vi "DUMMY.vi"() -> ()   [LabVIEW 2020]
uses:
  <vilib>/Waveform/WDTOps.llb/WDT Waveform Duration DBL.vi
  <vilib>/Waveform/WDTOps.llb/WDT Get Waveform Subset DBL.vi
  <vilib>/measure/mamon.llb/Trigger Detection for 1 Channel.vi
  <vilib>/measure/NI_MAPro.lvlib
  <vilib>/measure/mascope.llb/Transition Measurements 1 chan.vi
panel:
  out "error out":errorcluster
  out "file path (OUT)":path
  in  "Request #":string
  in  "Project #":string
  in  "TEST #":string
  out "DONE Tdon":bool
  in  "Decision ?":bool
  out "Tdon (ns) (after filter)":dbl
  out "Cursor a : Channel 2 (after filter)":dbl
  out "Cursor a : Channel 1 (after filter)":dbl
  in  "ICE":dbl
  in  "VGE":dbl
  out "10% Vge (Theory)":dbl
  out "10% Ice (Theory)":dbl
  out "measurement info (CH2) \n(after filter)":T1 {"ref levels"."ref units" items=["absolute", "relative"]; "ref levels"."high ref level" format="%.2p"; "ref levels"."low ref level" format="%.2p"; "ref levels"."mid ref level" format="%.2p"; "end time" format="%.6e"; "start time" format="%.6e"}
  in  "reference  levels (CH2 initialize) (after filter)":T2={"high ref level"=90.0, "mid ref level"=50.0, "low ref level"=10.0, "ref units"=1} {"ref units" items=["absolute", "percent"]; "high ref level" format="%0.2f"; "low ref level" format="%0.2f"; "mid ref level" format="%0.2f"}
  out "measurement info (CH1) \n(after filter)":T1 {"ref levels"."ref units" items=["absolute", "relative"]; "ref levels"."high ref level" format="%.2p"; "ref levels"."low ref level" format="%.2p"; "ref levels"."mid ref level" format="%.2p"; "end time" format="%.6e"; "start time" format="%.6e"}
  in  "reference  levels (CH1 initialize) (after filter)":T2={"high ref level"=90.0, "mid ref level"=50.0, "low ref level"=10.0, "ref units"=1} {"ref units" items=["absolute", "percent"]; "high ref level" format="%0.2f"; "low ref level" format="%0.2f"; "mid ref level" format="%0.2f"}
  out "Waveform Graph":waveform(dbl)[](graph)
  out "Tdon after Noise Filter":waveform(dbl)[](graph) caption="Tdon (ns)"
  in  "error in (no error)":errorcluster
  in  "file path (IN)":path
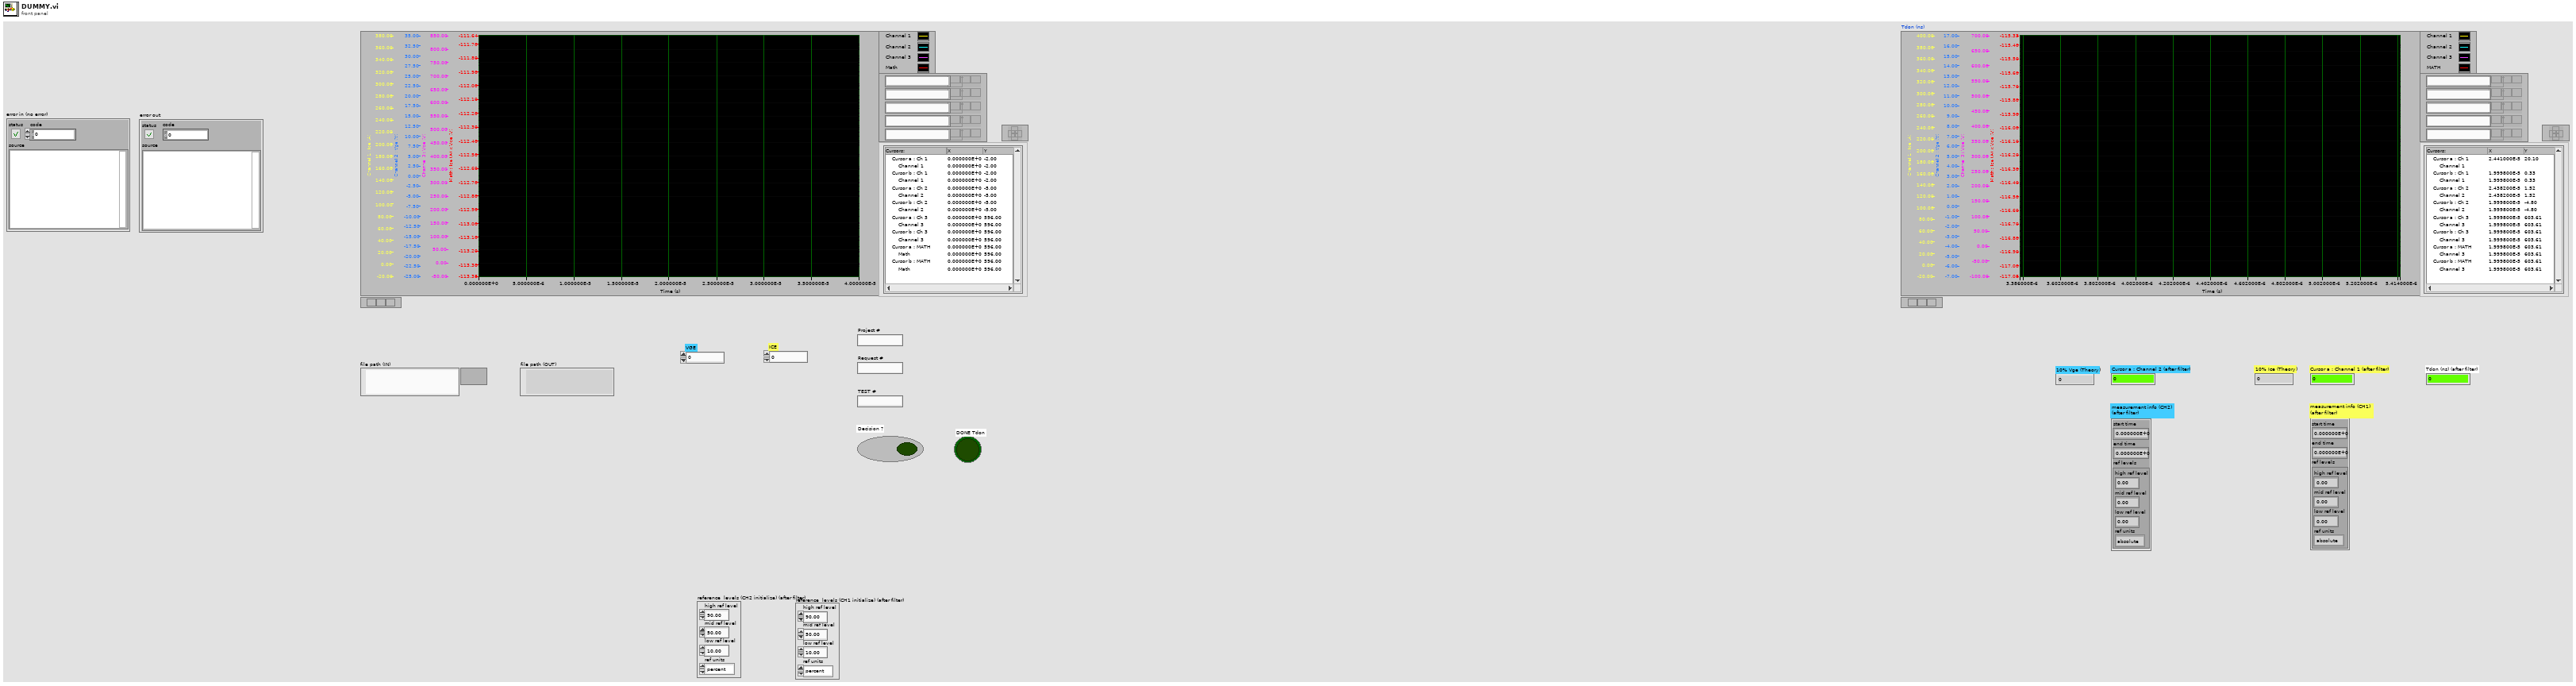
[diagram p1: front panel]
types:
  T1 = cluster{"start time":dbl, "end time":dbl, "ref levels":cluster{"high ref level":dbl, "mid ref level":dbl, "low ref level":dbl, "ref units":u16}}
  T2 = cluster{"high ref level":dbl, "mid ref level":dbl, "low ref level":dbl, "ref units":u16}
  T3 = enum32{"Invalid", "Standard", "Closed", "Hidden", "Minimized", "Maximized"}
  T4 = typedef "imagedata.ctl" = cluster{"image type":i32, "image depth":i32, "image":u8[], "mask":u8[], "colors":u32[], "Rectangle":cluster{"left":i16, "top":i16, "right":i16, "bottom":i16}}
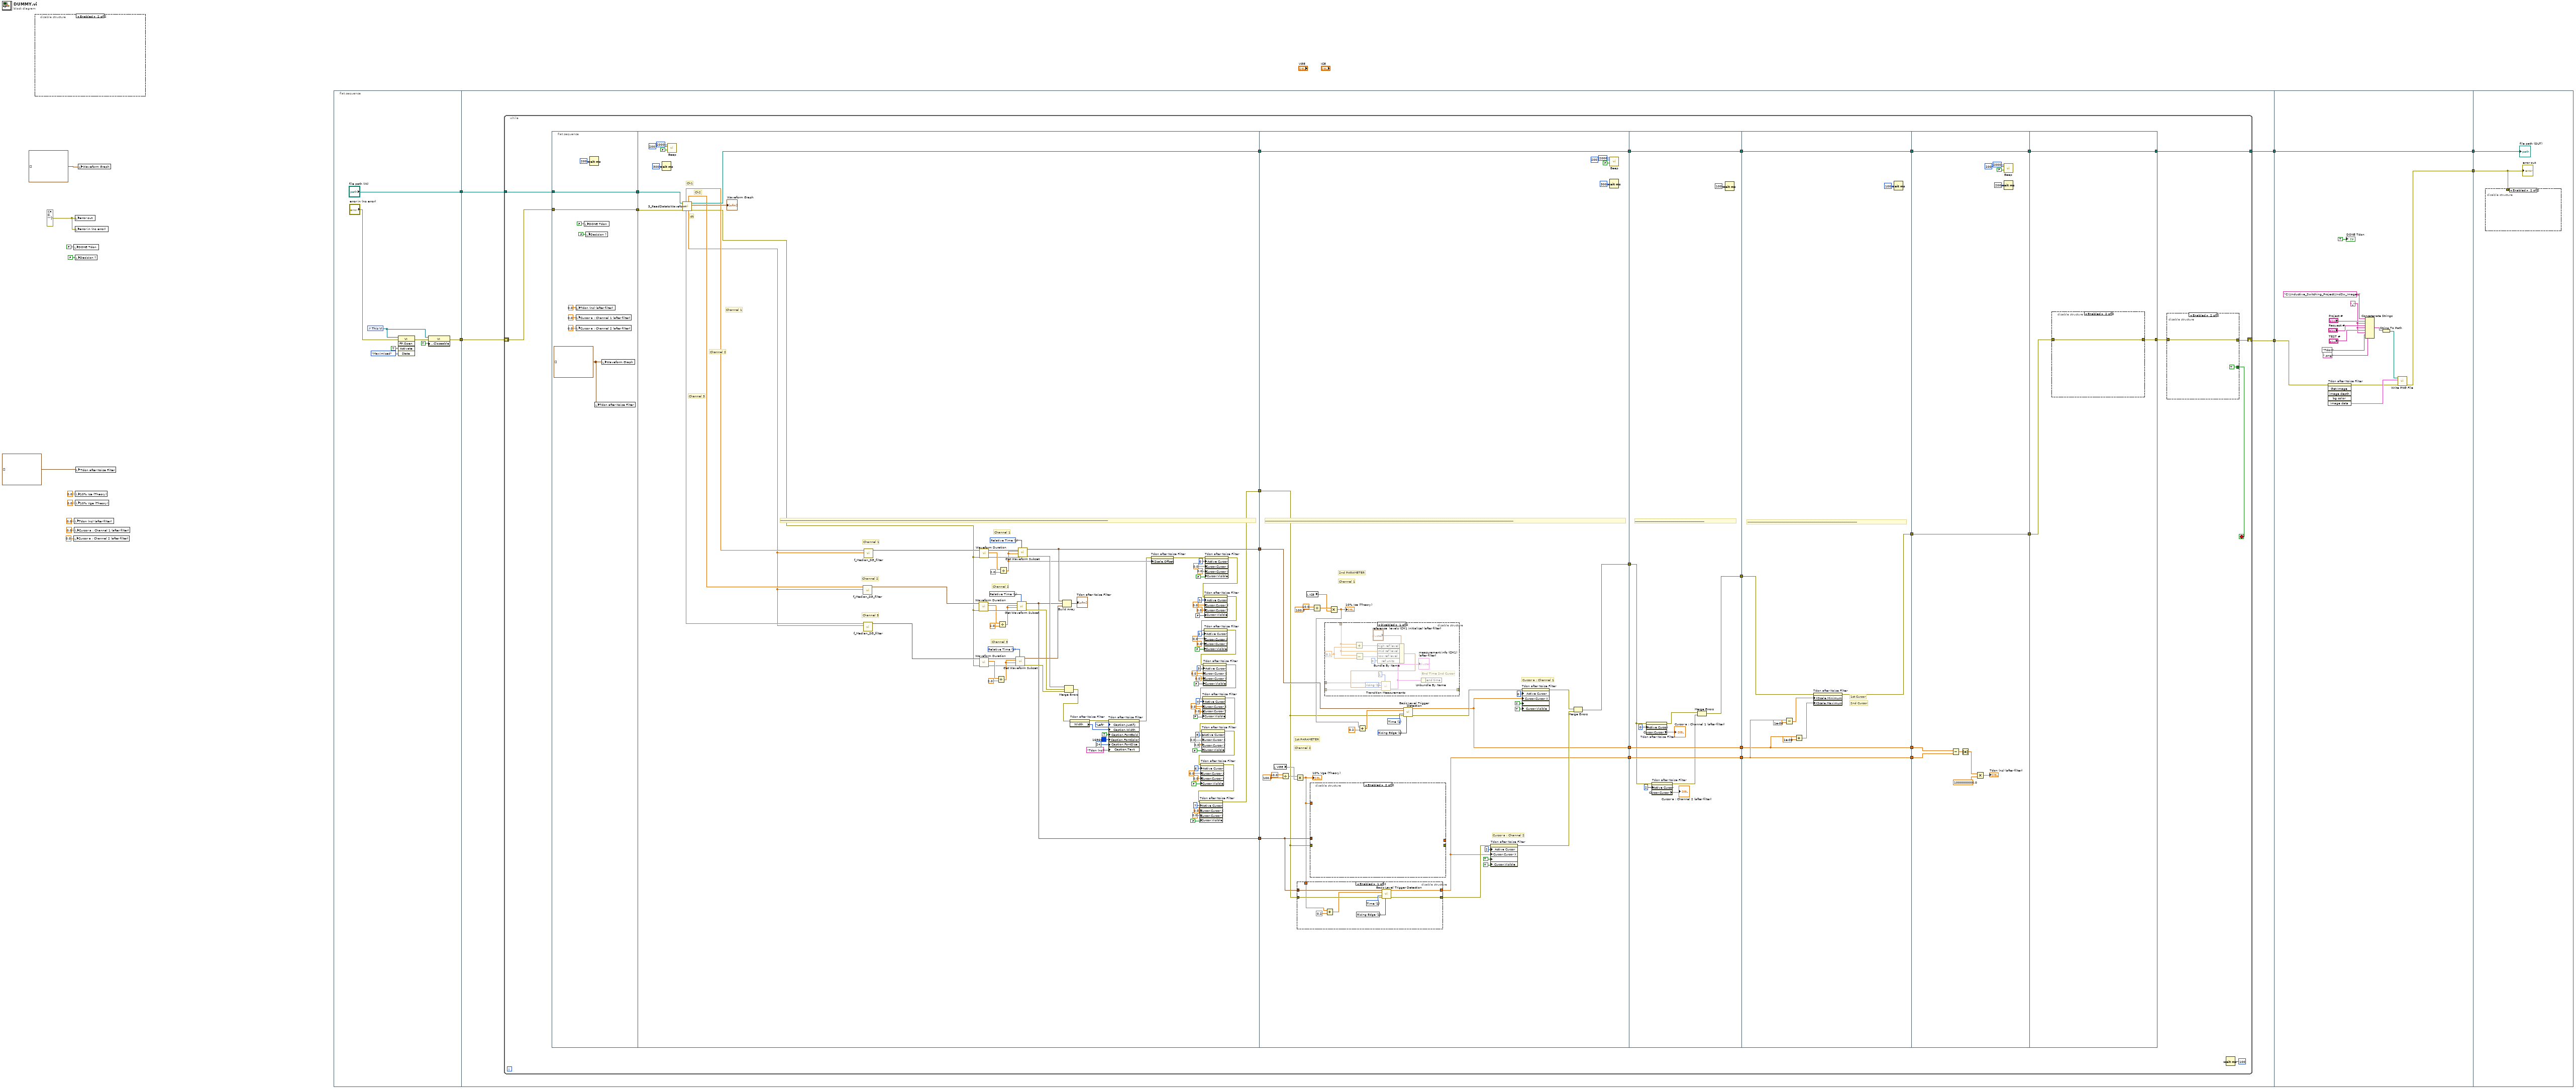
[diagram p0: block diagram]
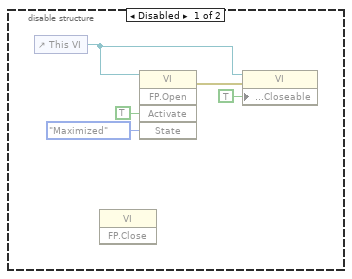
[diagram p2: hidden frame]
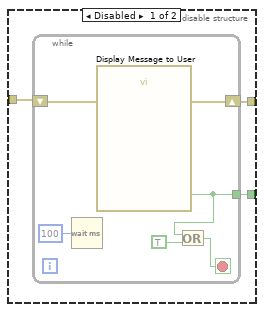
[diagram p3: hidden frame]
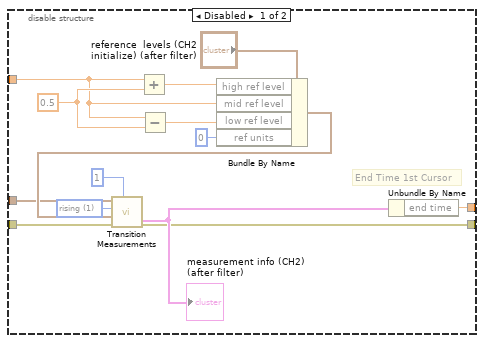
[diagram p6: hidden frame]
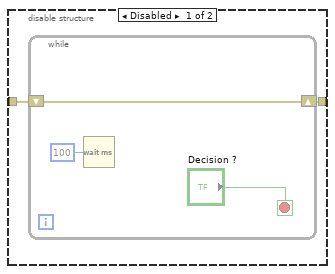
[diagram p7: hidden frame]
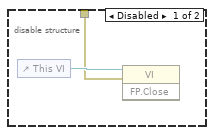
[diagram p8: hidden frame]
diagram:
  w9 = errorcluster {"status"=FALSE, "code"=0, "source"=""} ("error out")
  n1 = disable-structure shown="Enabled" {
    frame Disabled {
      n2 = control-ref of="This VI"() -> (w18:refnum<vi>)
      n3 = invoke class="VI" method="FP.Close"() -> (reference=w17:refnum<vi>)  [unwired: 2 in, 3 out]
      n4 = invoke class="VI" method="FP.Open"(reference=w18, "Activate"=TRUE ("Activate?"), "State"=T3."Maximized") -> (error in=w21:errorcluster, error out=w19:errorcluster)  [unwired: 1 in, 4 out]
      n5 = property class="VI"(reference=w18, error in=w19, "Front Panel.Closeable"=TRUE ("Front Panel Window:Closeable")) -> ()  [unwired: 2 out]
    }
    frame Enabled {
    }
  }
  n6 = local write "DONE Tdon"(FALSE ("DONE Tdon")) -> ()
  n7 = local write "Cursor a : Channel 2 (after filter)"(0.0 ("Cursor a : Channel 2 (after filter)")) -> ()
  n8 = local write "Tdon (ns) (after filter)"(0.0 ("Tdon (ns) (after filter)")) -> ()
  n9 = local write "Cursor a : Channel 1 (after filter)"(0.0 ("Cursor a : Channel 1 (after filter)")) -> ()
  n10 = local write "error out"(w9) -> ()
  n11 = local write "error in (no error)"(w9) -> ()
  n12 = local write "Decision ?"(FALSE ("Decision ?")) -> ()
  n13 = local write "10% Ice (Theory)"(0.0 ("10% Ice (Theory)")) -> ()
  n14 = local write "10% Vge (Theory)"(0.0 ("10% Vge (Theory)")) -> ()
  n15 = local write "Tdon after Noise Filter"(waveform(dbl)[] [] ("Tdon after Noise Filter")) -> ()
  n16 = local write "Waveform Graph"(waveform(dbl)[] [] ("Waveform Graph")) -> ()
  n17 = flat-sequence {
    tunnel: ["file path (IN)"] -> w16
    tunnel: [w26] -> w15
    tunnel: [w34] -> w14
    tunnel: [w33] -> w13
    tunnel: w16 -> [w35]
    tunnel: w15 -> [w32]
    tunnel: w14 -> [w289]
    tunnel: [w292] -> w12
    tunnel: [w291] -> w11
    tunnel: w13 -> [w291]
    tunnel: w12 -> [w303]
    tunnel: w11 -> [w304]
    frame #0 {
      n18 = control-ref of="This VI"() -> (w30:refnum<vi>)
      n19 = invoke class="VI" method="FP.Open"(reference=w30, error in="error in (no error)", "Activate"=TRUE ("Activate?"), "State"=T3."Maximized") -> (error out=w31:errorcluster)  [unwired: 1 in, 4 out]
      n20 = property class="VI"(reference=w30, error in=w31, "Front Panel.Closeable"=TRUE ("Front Panel Window:Closeable")) -> (error out=w26:errorcluster)  [unwired: 1 out]
    }
    frame #1 {
      n21 = while {
        tunnel: w35 -> [w58]
        shift-right: [w38] -> w34
        shift-left: w32 -> [w56]
        tunnel: [w54] -> w33
        stop <- w37 stop-if-true
        n22 = flat-sequence {
          tunnel: [w81] -> w62
          tunnel: [w82] -> w61
          tunnel: w58 -> [w82]
          tunnel: w56 -> [w81]
          tunnel: w62 -> [w173]
          tunnel: w61 -> [w171]
          tunnel: [w167] -> w60
          tunnel: [w141] -> w50
          tunnel: [w86] -> w49
          tunnel: [w83] -> w36
          tunnel: w60 -> [w205]
          tunnel: [w205] -> w53
          tunnel: w50 -> [w183]
          tunnel: w49 -> [w177]
          tunnel: [w188] -> w48
          tunnel: [w181] -> w47
          tunnel: [w174] -> w46
          tunnel: w36 -> [w187]
          tunnel: w53 -> [w256]
          tunnel: [w256] -> w52
          tunnel: w48 -> [w245]
          tunnel: w47 -> [w253]
          tunnel: w46 -> [w252]
          tunnel: [w253] -> w45
          tunnel: [w252] -> w44
          tunnel: [w246] -> w43
          tunnel: w52 -> [w266]
          tunnel: [w266] -> w59
          tunnel: w45 -> [w259]
          tunnel: w44 -> [w262]
          tunnel: w43 -> [w257]
          tunnel: [w262] -> w42
          tunnel: [w259] -> w41
          tunnel: [w258] -> w39
          tunnel: w59 -> [w275]
          tunnel: [w275] -> w55
          tunnel: w42 -> [w269]
          tunnel: w41 -> [w270]
          tunnel: [w267] -> w40
          tunnel: w39 -> [w267]
          tunnel: [w279] -> w51
          tunnel: w55 -> [w281]
          tunnel: [w281] -> w54
          tunnel: w40 -> [w280]
          frame #0 {
            w77 = waveform(dbl)[] [] ("Waveform Graph")
            n23 = local write "Tdon (ns) (after filter)"(0.0 ("Tdon (ns) (after filter)")) -> ()
            n24 = local write "Cursor a : Channel 1 (after filter)"(0.0 ("Cursor a : Channel 1 (after filter)")) -> ()
            n25 = local write "Cursor a : Channel 2 (after filter)"(0.0 ("Cursor a : Channel 2 (after filter)")) -> ()
            n26 = local write "DONE Tdon"(FALSE ("DONE Tdon")) -> ()
            n27 = local write "Decision ?"(FALSE ("Decision ?")) -> ()
            n28 = Wait (ms)(milliseconds to wait=u32 200) -> ()  [unwired: 1 out]
            n29 = local write "Tdon after Noise Filter"(w77) -> ()
            n30 = local write "Waveform Graph"(w77) -> ()
          }
          frame #1 {
            w162 = u16 1 items=["Samples", "Relative Time"] ("start/duration format")
            w151 = u16 1 items=["Samples", "Relative Time"] ("start/duration format")
            w150 = u16 1 items=["Samples", "Relative Time"] ("start/duration format")
            # "--------------------------------------------------------------------------------------------------------------------------------------------------------------------------------------------------------------------------------------------------------------------------------------------------------------------------------------"
            # "Channel 1"
            # "Channel 3"
            # "Channel 2"
            # "Channel 3"
            # "Channel 2"
            # "Channel 1"
            # "Channel 3"
            # "Channel 2"
            # "Channel 1"
            # "dt"
            # "Ch2"
            # "Ch1"
            n31 = Wait (ms)(milliseconds to wait=u32 300) -> ()  [unwired: 1 out]
            n32 = call <vilib>:"Beep.vi"("use system alert? (T)"=FALSE, "duration (msec)"=u32 200, "frequency (Hz)"=u32 2000) -> ()  [unwired: 9 in]
            n33 = call "3_ReadDatatoWaveform.vi"("error in (no error)"=w173, "file path (IN)"=w171) -> ("error out"=w84:errorcluster, "Waveform Graph"=→"Waveform Graph":waveform(dbl)[], "file path (OUT)"=w167:path, "dt"=w85:dbl, "Ch 2 Data"=w164:dbl[], "Ch 3 Data"=w163:dbl[], "Ch 1 Data"=w165:dbl[])  [unwired: 3 in]
            n34 = call "f_Median_SG_filter.vi"("dt"=w85, "Y"=w164) -> ("output waveform"=w144:waveform(dbl))  [unwired: 9 in]
            n35 = call "f_Median_SG_filter.vi"("dt"=w85, "Y"=w163) -> ("output waveform"=w143:waveform(dbl))  [unwired: 9 in]
            n36 = call "f_Median_SG_filter.vi"("dt"=w85, "Y"=w165) -> ("output waveform"=w145:waveform(dbl))  [unwired: 9 in]
            n37 = call-poly <vilib>:"Waveform Duration.vi"("error in (no error)"=w84, "waveform in"=w144) -> ("error out"=w156:errorcluster, "duration"=w153:dbl, "waveform out"=w155:waveform(dbl))  [unwired: 7 in]
            n38 = call-poly <vilib>:"Waveform Duration.vi"("error in (no error)"=w84, "waveform in"=w143) -> ("error out"=w157:errorcluster, "duration"=w160:dbl, "waveform out"=w158:waveform(dbl))  [unwired: 7 in]
            n39 = call-poly <vilib>:"Waveform Duration.vi"("error in (no error)"=w84, "waveform in"=w145) -> ("error out"=w146:errorcluster, "duration"=w149:dbl, "waveform out"=w147:waveform(dbl))  [unwired: 7 in]
            n40 = Divide(x=w160, y=2.0) -> (x/y=w161:dbl)
            n41 = Divide(x=w153, y=2.0) -> (x/y=w152:dbl)
            n42 = Divide(x=w149, y=2.0) -> (x/y=w128:dbl)
            n43 = call-poly <vilib>:"Get Waveform Subset.vi"("start/duration format"=w162, "error in (no error)"=w157, "duration"=w161, "start samples/time"=w161, "waveform in"=w158) -> ("error out"=w137:errorcluster, "waveform out"=w140:waveform(dbl))  [unwired: 1 in, 2 out]
            n44 = call-poly <vilib>:"Get Waveform Subset.vi"("start/duration format"=w151, "error in (no error)"=w156, "duration"=w152, "start samples/time"=w152, "waveform in"=w155) -> ("error out"=w138:errorcluster, "waveform out"=w83:waveform(dbl))  [unwired: 1 in, 2 out]
            n45 = call-poly <vilib>:"Get Waveform Subset.vi"("start/duration format"=w150, "error in (no error)"=w146, "duration"=w128, "start samples/time"=w128, "waveform in"=w147) -> ("error out"=w139:errorcluster, "waveform out"=w141:waveform(dbl))  [unwired: 1 in, 2 out]
            n46 = Build Array(w141, w83, w140) -> (→"Tdon after Noise Filter":waveform(dbl)[])
            n47 = Merge Errors(w139, w138, w137) -> (w136:errorcluster)
            n48 = property on="Tdon after Noise Filter" class="WFGraph (strict)"(error in=w136) -> (error out=w130:errorcluster, "Width"=w129:u32)  [unwired: 1 in, 1 out]
            n49 = property on="Tdon after Noise Filter" class="WFGraph (strict)"(error in=w130, "Caption.Justify"=enum16{"Left", "Center", "Right"}."Left" ("Caption.Justification"), "Caption.Width"=w129, "Caption.FontBold"=TRUE ("Caption.Font:Bold"), "Caption.FontColor"=u32 16860 ("Caption.Font:Color"), "Caption.FontSize"=u32 24 ("Caption.Font:Size"), "Caption.Text"="Tdon (ns)") -> (error out=w127:errorcluster)  [unwired: 1 in, 1 out]
            n50 = property on="Tdon after Noise Filter" class="WFGraph (strict)"(error in=w127, "XScale.Offset"=w128) -> (error out=w94:errorcluster)  [unwired: 1 in, 1 out]
            n51 = property on="Tdon after Noise Filter" class="WFGraph (strict)"(error in=w94, "Active Cursor"=u32 0, "Cursor.Cursor X"=0.0 ("Cursor.Cursor Position:Cursor X"), "Cursor.Cursor Y"=0.0 ("Cursor.Cursor Position:Cursor Y"), "Cursor.Visible"=FALSE) -> (error out=w93:errorcluster)  [unwired: 1 in, 1 out]
            n52 = property on="Tdon after Noise Filter" class="WFGraph (strict)"(error in=w93, "Active Cursor"=u32 1, "Cursor.Cursor X"=0.0 ("Cursor.Cursor Position:Cursor X"), "Cursor.Cursor Y"=0.0 ("Cursor.Cursor Position:Cursor Y"), "Cursor.Visible"=FALSE) -> (error out=w92:errorcluster)  [unwired: 1 in, 1 out]
            n53 = property on="Tdon after Noise Filter" class="WFGraph (strict)"(error in=w92, "Active Cursor"=u32 2, "Cursor.Cursor X"=0.0 ("Cursor.Cursor Position:Cursor X"), "Cursor.Cursor Y"=0.0 ("Cursor.Cursor Position:Cursor Y"), "Cursor.Visible"=FALSE) -> (error out=w91:errorcluster)  [unwired: 1 in, 1 out]
            n54 = property on="Tdon after Noise Filter" class="WFGraph (strict)"(error in=w91, "Active Cursor"=u32 3, "Cursor.Cursor X"=0.0 ("Cursor.Cursor Position:Cursor X"), "Cursor.Cursor Y"=0.0 ("Cursor.Cursor Position:Cursor Y"), "Cursor.Visible"=FALSE) -> (error out=w90:errorcluster)  [unwired: 1 in, 1 out]
            n55 = property on="Tdon after Noise Filter" class="WFGraph (strict)"(error in=w90, "Active Cursor"=u32 4, "Cursor.Cursor X"=0.0 ("Cursor.Cursor Position:Cursor X"), "Cursor.Cursor Y"=0.0 ("Cursor.Cursor Position:Cursor Y"), "Cursor.Visible"=FALSE) -> (error out=w89:errorcluster)  [unwired: 1 in, 1 out]
            n56 = property on="Tdon after Noise Filter" class="WFGraph (strict)"(error in=w89, "Active Cursor"=u32 5, "Cursor.Cursor X"=0.0 ("Cursor.Cursor Position:Cursor X"), "Cursor.Cursor Y"=0.0 ("Cursor.Cursor Position:Cursor Y"), "Cursor.Visible"=FALSE) -> (error out=w88:errorcluster)  [unwired: 1 in, 1 out]
            n57 = property on="Tdon after Noise Filter" class="WFGraph (strict)"(error in=w88, "Active Cursor"=u32 6, "Cursor.Cursor X"=0.0 ("Cursor.Cursor Position:Cursor X"), "Cursor.Cursor Y"=0.0 ("Cursor.Cursor Position:Cursor Y"), "Cursor.Visible"=FALSE) -> (error out=w87:errorcluster)  [unwired: 1 in, 1 out]
            n58 = property on="Tdon after Noise Filter" class="WFGraph (strict)"(error in=w87, "Active Cursor"=u32 7, "Cursor.Cursor X"=0.0 ("Cursor.Cursor Position:Cursor X"), "Cursor.Cursor Y"=0.0 ("Cursor.Cursor Position:Cursor Y"), "Cursor.Visible"=FALSE) -> (error out=w86:errorcluster)  [unwired: 1 in, 1 out]
          }
          frame #2 {
            w184 = u16 1 items=["Falling Edge", "Rising Edge"] ("trigger slope")
            w185 = u16 1 items=["Index", "Time"] ("location mode")
            # "Cursor a : Channel 1"
            # "2nd PARAMETER"
            # "Channel 1"
            # "Cursor a : Channel 2"
            # "1st PARAMETER"
            # "Channel 2"
            # "-------------------------------------------------------------------------------------------------------------------------------------------------------------------------------------------------------------------------------------------------------"
            n59 = local read "VGE"() -> (w186:dbl)
            n60 = Divide(x=10.0, y=100.0) -> (x/y=w202:dbl)
            n61 = Multiply(x=w202, y=w186) -> (x*y=w176:dbl)
            "10% Vge (Theory)" <- w176
            n62 = disable-structure shown="Enabled" {
              disable-tunnel: [w217 _] -> w174
              disable-tunnel: w187 -> [w216 _]
              disable-tunnel: [w215 _] -> w175
              disable-tunnel: w177 -> [w212 _]
              disable-tunnel: w176 -> [w210 _]
              frame Enabled {
                w213 = u16 1 items=["Falling Edge", "Rising Edge"] ("trigger slope")
                w214 = u16 1 items=["Index", "Time"] ("location mode")
                n63 = Add(x=w210, y=0.2) -> (x+y=w209:dbl)
                n64 = call-poly <vilib>:"Basic Level Trigger Detection.vi"("signal in"=w216, "level"=w209, "location mode"=w214, "error in (no error)"=w212, "trigger slope"=w213) -> ("trigger location"=w217:dbl, "error out"=w215:errorcluster)  [unwired: 8 in, 1 out]
              }
              frame Disabled {
              }
            }
            n65 = local read "ICE"() -> (w194:dbl)
            n66 = disable-structure shown="Enabled" {
              disable-tunnel: w187 -> [w237 _]
              disable-tunnel: w177 -> [w234 _]
              disable-tunnel: [w233 _] -> _
              disable-tunnel: w176 -> [w232 _]
              disable-tunnel: [w231 _] -> _
              frame Disabled {
                w236 = 0.5 ("y")
                w239 = u16 1 items=["falling", "rising"] ("polarity (rising)")
                # "End Time 1st Cursor"
                n67 = Add(x=w232, y=w236) -> (x+y=w240:dbl)
                n68 = Subtract(x=w232, y=w236) -> (x-y=w241:dbl)
                n69 = Bundle By Name(cluster="reference  levels (CH2 initialize) (after filter)", "high ref level"=w240, "mid ref level"=w232, "low ref level"=w241, "ref units"=u16 0) -> (w244:T2)
                n70 = call-poly <vilib>:"Transition Measurements.vi"("edge number (1)"=1, "error in (no error)"=w234, "reference levels"=w244, "polarity (rising)"=w239, "signal in"=w237) -> ("error out"=w233:errorcluster, "measurement info"=w235:T1)  [unwired: 1 in, 4 out]
                "measurement info (CH2) \n(after filter)" <- w235
                n71 = Unbundle By Name(w235) -> ("end time"=w231:dbl)
              }
              frame Enabled {
              }
            }
            n72 = Divide(x=10.0, y=100.0) -> (x/y=w195:dbl)
            n73 = disable-structure shown="Disabled" {
              disable-tunnel: _ -> [w224 _]
              disable-tunnel: _ -> [w220 _]
              disable-tunnel: [w219 _] -> _
              disable-tunnel: _ -> [w218 _]
              frame Disabled {
                w223 = 0.1 ("y")
                w225 = u16 1 items=["falling", "rising"] ("polarity (rising)")
                # "End Time 2nd Cursor"
                n74 = Add(x=w220, y=w223) -> (x+y=w226:dbl)
                n75 = Subtract(x=w220, y=w223) -> (x-y=w227:dbl)
                n76 = Bundle By Name(cluster="reference  levels (CH1 initialize) (after filter)", "high ref level"=w226, "mid ref level"=w220, "low ref level"=w227, "ref units"=u16 0) -> (w230:T2)
                n77 = call-poly <vilib>:"Transition Measurements.vi"("edge number (1)"=1, "error in (no error)"=w218, "reference levels"=w230, "polarity (rising)"=w225, "signal in"=w224) -> ("error out"=w219:errorcluster, "measurement info"=w221:T1)  [unwired: 1 in, 4 out]
                "measurement info (CH1) \n(after filter)" <- w221
                n78 = Unbundle By Name(w221) -> ()  [unwired: 1 out]
              }
              frame Enabled {
              }
            }
            n79 = Multiply(x=w195, y=w194) -> (x*y=w179:dbl)
            "10% Ice (Theory)" <- w179
            n80 = Add(x=w179, y=0.2) -> (x+y=w178:dbl)
            n81 = call-poly <vilib>:"Basic Level Trigger Detection.vi"("signal in"=w183, "level"=w178, "location mode"=w185, "error in (no error)"=w177, "trigger slope"=w184) -> ("trigger location"=w181:dbl, "error out"=w182:errorcluster)  [unwired: 8 in, 1 out]
            n82 = property on="Tdon after Noise Filter" class="WFGraph (strict)"(error in=w175, "Active Cursor"=u32 2, "Cursor.Cursor X"=w174, "Cursor.Cursor Name Visible"=TRUE, "Cursor.Visible"=TRUE) -> (error out=w190:errorcluster)  [unwired: 1 in, 1 out]
            n83 = property on="Tdon after Noise Filter" class="WFGraph (strict)"(error in=w182, "Active Cursor"=u32 0, "Cursor.Cursor X"=w181, "Cursor.Cursor Name Visible"=TRUE, "Cursor.Visible"=TRUE) -> (error out=w189:errorcluster)  [unwired: 1 in, 1 out]
            n84 = Merge Errors(w189, w190) -> (w188:errorcluster)
            n85 = call <vilib>:"Beep.vi"("use system alert? (T)"=FALSE, "duration (msec)"=u32 200, "frequency (Hz)"=u32 2000) -> ()  [unwired: 9 in]
            n86 = Wait (ms)(milliseconds to wait=u32 300) -> ()  [unwired: 1 out]
          }
          frame #3 {
            # "---------------------------------------------------------------------"
            n87 = property on="Tdon after Noise Filter" class="WFGraph (strict)"(error in=w245, "Active Cursor"=u32 0) -> (error out=w251:errorcluster, "Cursor.Cursor Y"=→"Cursor a : Channel 1 (after filter)":dbl)  [unwired: 1 in, 1 out]
            n88 = property on="Tdon after Noise Filter" class="WFGraph (strict)"(error in=w245, "Active Cursor"=u32 2) -> (error out=w250:errorcluster, "Cursor.Cursor Y"=→"Cursor a : Channel 2 (after filter)":dbl)  [unwired: 1 in, 1 out]
            n89 = Merge Errors(w251, w250) -> (w246:errorcluster)
            n90 = Wait (ms)(milliseconds to wait=u32 100) -> ()  [unwired: 1 out]
          }
          frame #4 {
            # "2nd Cursor"
            # "1st Cursor"
            # "-------------------------------------------------------------------------------------------------------------"
            n91 = Subtract(x=w262, y=1e-06) -> (x-y=w261:dbl)
            n92 = Add(x=w259, y=1e-06) -> (x+y=w260:dbl)
            n93 = property on="Tdon after Noise Filter" class="WFGraph (strict)"(error in=w257, "XScale.Minimum"=w261, "XScale.Maximum"=w260) -> (error out=w258:errorcluster)  [unwired: 1 in, 1 out]
            n94 = Wait (ms)(milliseconds to wait=u32 100) -> ()  [unwired: 1 out]
          }
          frame #5 {
            n95 = Subtract(x=w270, y=w269) -> (x-y=w272:dbl)
            n96 = Absolute Value(x=w272) -> (abs(x)=w273:dbl)
            n97 = Multiply(x=w273, y=1000000000.0) -> (x*y=→"Tdon (ns) (after filter)":dbl)
            n98 = call <vilib>:"Beep.vi"("use system alert? (T)"=FALSE, "duration (msec)"=u32 200, "frequency (Hz)"=u32 2000) -> ()  [unwired: 9 in]
            n99 = Wait (ms)(milliseconds to wait=u32 200) -> ()  [unwired: 1 out]
          }
          frame #6 {
            n100 = disable-structure shown="Enabled" {
              disable-tunnel: w280 -> [w283 w287]
              disable-tunnel: [w282 w287] -> w279
              frame Disabled {
                n101 = while {
                  shift-right: [w284] -> w282
                  shift-left: w283 -> [w284]
                  stop <- "Decision ?" stop-if-true
                  n102 = Wait (ms)(milliseconds to wait=u32 100) -> ()  [unwired: 1 out]
                }
              }
              frame Enabled {
              }
            }
          }
        }
        n103 = disable-structure shown="Enabled" {
          disable-tunnel: w51 -> [w65 w73]
          disable-tunnel: [w64 w73] -> w38
          disable-tunnel: [w63 TRUE ("NO")] -> w37
          frame Disabled {
            n104 = while {
              tunnel: [w67] -> w63
              shift-right: [w70] -> w64
              shift-left: w65 -> [w71]
              stop <- w69 stop-if-true
              n105 = Wait (ms)(milliseconds to wait=u32 100) -> ()  [unwired: 1 out]
              n106 = call "Display Message to User"("error in (no error)"=w71) -> ("error out"=w70:errorcluster, "NO"=w67:bool)  [unwired: 9 in]
              n107 = Or(x=w67, y=TRUE) -> (x .or. y?=w69:bool)
            }
          }
          frame Enabled {
          }
        }
        n108 = Wait (ms)(milliseconds to wait=u32 100) -> ()  [unwired: 1 out]
      }
    }
    frame #2 {
      w295 = "_"
      n109 = invoke on="Tdon after Noise Filter" class="WFGraph (strict)" method="Get Image"(error in=w289) -> (error out=w288:errorcluster, "image data"=w290:T4)  [unwired: 5 in, 4 out]
      n110 = Concatenate Strings("C:\\Inductive_Switching_Project\\IndSw_Image\\" ("string"), "Project #", w295, "Request #", w295, "TEST #", w295, "Tdon" ("string"), ".png" ("string")) -> (w300:string)
      n111 = String To Path(string=w300) -> (path=w299:path)
      n112 = call <vilib>:"Write PNG File.vi"("error in (no error)"=w288, "image data"=w290, "path to PNG file"=w299) -> ("error out"=w292:errorcluster)  [unwired: 7 in, 1 out]
      "DONE Tdon" <- TRUE ("DONE Tdon")
    }
    frame #3 {
      n113 = disable-structure shown="Enabled" {
        disable-tunnel: w303 -> [w305 _]
        frame Disabled {
          n114 = control-ref of="This VI"() -> (w306:refnum<vi>)
          n115 = invoke class="VI" method="FP.Close"(reference=w306, error in=w305) -> ()  [unwired: 1 in, 3 out]
        }
        frame Enabled {
        }
      }
      "error out" <- w303
      "file path (OUT)" <- w304
    }
  }
